vi "Pre Launch Init.vi"(11 "Counter in":refnum<class "Counter.lvclass">) -> (0 "error out":errorcluster, 3 "Counter out":refnum<class "Counter.lvclass">)   [LabVIEW 2020, in "Counter.lvlib" / "Counter.lvclass"]
doc: "(<B>Filename</B>: Actor Framework.lvlib:Actor.lvclass:Pre Launch Init.vi)\n\nDefines behavior that occurs after the Launch Nested Actor method is invoked but before the actor's Actor Core method begins running.\n\nBy default, this method does nothing. A descendant class may override it to define behavior."
uses:
  Counter.lvclass
  Counter.lvclass/Counter.ctl
  <vilib>/ActorFramework/Actor/Actor.lvclass
  Counter.lvlib
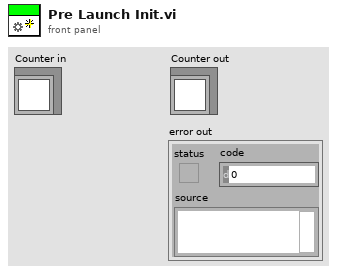
[diagram p1: front panel]
types:
  T1 = cluster{"Exit Event":refnum<user-event>, "Start/Stop Event":refnum<user-event>, "Limit Change Event":refnum<user-event>}
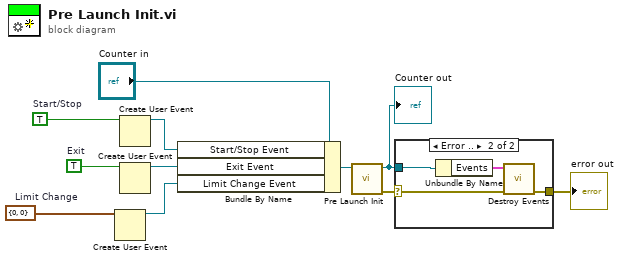
[diagram p0: block diagram]
diagram:
  w8 = cluster{"Upper Limit":u8, "Lower Limit":u8} {"Upper Limit"=0, "Lower Limit"=0}  # Limit Change
  w9 = TRUE  # Exit
  w10 = TRUE  # Start/Stop
  n1 = Create User Event(user event datatype=w8) -> (user event=w4:refnum<user-event>)  [unwired: 1 in, 1 out]
  n2 = Create User Event(user event datatype=w10) -> (user event=w6:refnum<user-event>)  [unwired: 1 in, 1 out]
  n3 = Create User Event(user event datatype=w9) -> (user event=w5:refnum<user-event>)  [unwired: 1 in, 1 out]
  n4 = Bundle By Name(cluster="Counter in", "Start/Stop Event"=w6, "Exit Event"=w5, "Limit Change Event"=w4) -> (w7:refnum<class "Counter.lvclass">)
  n5 = call-parent "Pre Launch Init.vi"("Actor in"=w7) -> ("error out"=w3:errorcluster, "Actor out"=w1:refnum<class "Counter.lvclass">)  [unwired: 9 in]
  "Counter out" <- w1
  n6 = case shown="Error .." w3 {
    selector: w3 -> [w12 w14]
    tunnel: [w12 w13] -> w2
    tunnel: w1 -> [_ w16]
    frame No Error {
    }
    frame Error {
      n7 = Unbundle By Name(w16) -> ("Events"=w15:T1)
      n8 = call "Destroy Events.vi"("error in"=w14, "Events"=w15) -> ("error out"=w13:errorcluster)  [unwired: 9 in]
    }
  }
  "error out" <- w2
